vi "Acnetize to ACNET Devices.vi"(8 "error in (no error)":errorcluster, 11 "Acnetize Configuration":string) -> (0 "error out":errorcluster, 3 "ACNET Devices":refnum<class "ACNET Devices.lvclass">)   [LabVIEW 2013]
uses:
  ACNET Monitor/ACNET Devices.lvclass
  ACNET Monitor/ACNET Device.lvclass
  <vilib>/wsapi/NI_WebServices.lvlib
panel:
  out "Array":T1(array[cluster])
  out "subarray":string[](array[string])
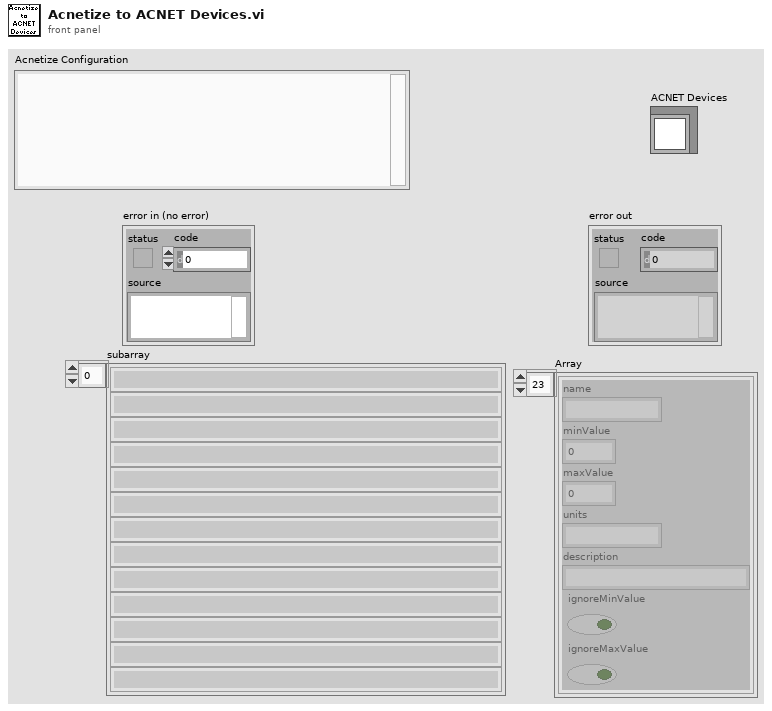
[diagram p1: front panel]
types:
  T1 = cluster{"name":string, "minValue":dbl, "maxValue":dbl, "units":string, "description":string, "ignoreMinValue":bool, "ignoreMaxValue":bool}[]
  T2 = cluster{"name":string, "minValue":dbl, "maxValue":dbl, "units":string, "description":string, "ignoreMinValue":bool, "ignoreMaxValue":bool}
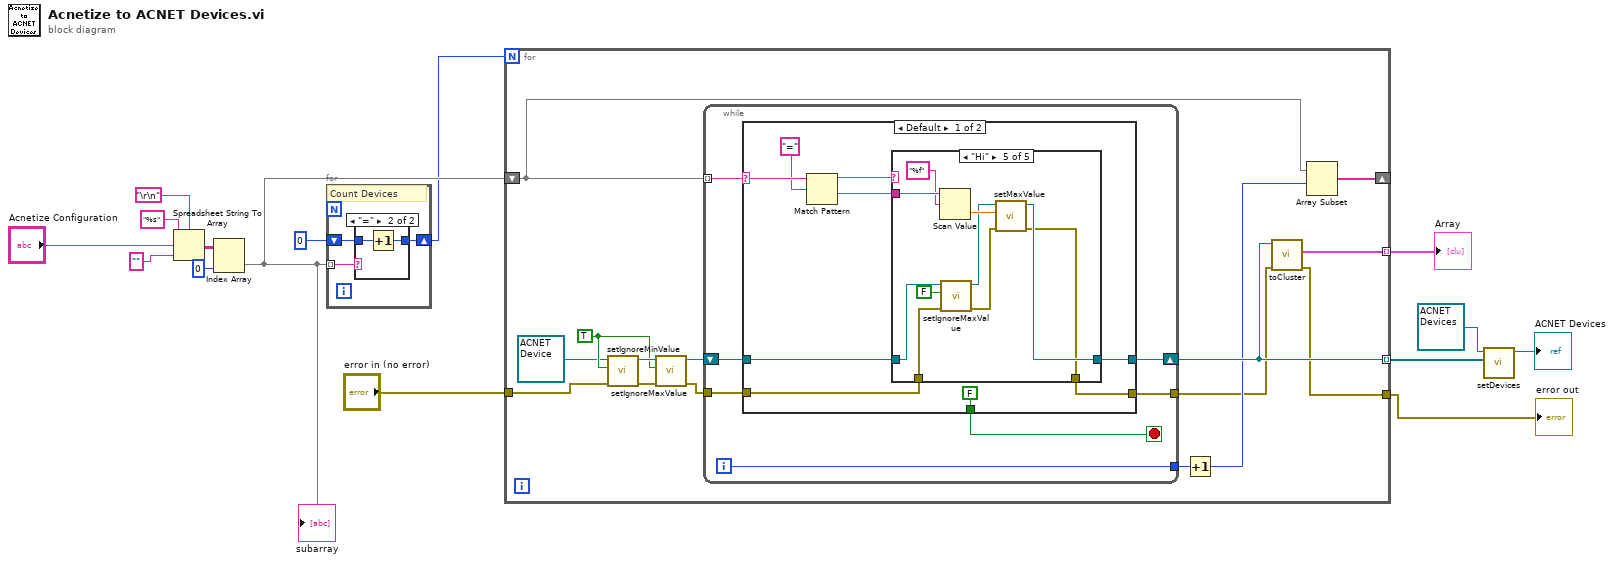
[diagram p0: block diagram]
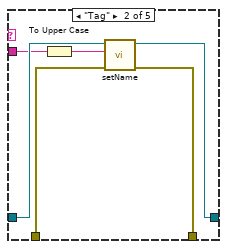
[diagram p3: hidden frame]
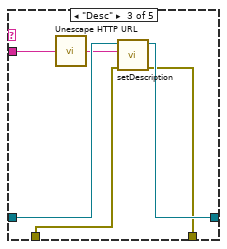
[diagram p4: hidden frame]
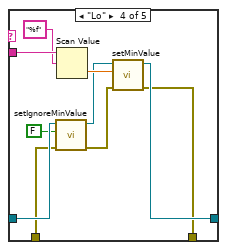
[diagram p5: hidden frame]
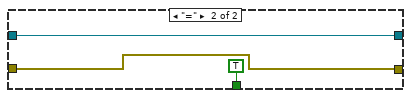
[diagram p6: hidden frame]
diagram:
  n1 = Spreadsheet String To Array(delimiter (Tab)="\r\n", format string="%s", spreadsheet string="Acnetize Configuration", array type (2D Dbl)="") -> (array=w11:string[][])
  n2 = Index Array(array=w11, index (col)=0 ("disabled index (col)")) -> (element=w9:string[])  [unwired: 1 in]
  "subarray" <- w9
  n3 = for {
    tunnel: w9 -> [w18] mode=indexing
    shift-right: [w16] -> w3
    shift-left: 0 -> [w17]
    # "Count Devices"
    n4 = case shown="\"=\"" w18 {
      tunnel: w17 -> [w19 w21]
      tunnel: [w19 w20] -> w16
      frame Default {
      }
      frame "=" {
        n5 = Increment(x=w21) -> (x+1=w20:i32)
      }
    }
  }
  n6 = for {
    N: w3 -> [_]
    tunnel: [w36] -> w7 mode=indexing
    tunnel: [w35] -> w4 mode=indexing
    shift-right: [w31] -> _
    shift-left: w9 -> [w32]
    tunnel: "error in (no error)" -> [w24]
    tunnel: [w29] -> w1
    w26 = TRUE ("ignoreMinValue")
    n7 = call-dynamic "setIgnoreMinValue.vi"("error in (no error)"=w24, "ignoreMinValue"=w26, "ACNET Device in"=refnum<class "ACNET Device.lvclass"> refnum ("ACNET Device.lvclass")) -> ("error out"=w28:errorcluster, "ACNET Device out"=w27:refnum<class "ACNET Device.lvclass">)  [unwired: 7 in]
    n8 = call-dynamic "setIgnoreMaxValue.vi"("error in (no error)"=w28, "ignoreMaxValue"=w26, "ACNET Device in"=w27) -> ("error out"=w23:errorcluster, "ACNET Device out"=w22:refnum<class "ACNET Device.lvclass">)  [unwired: 7 in]
    n9 = while {
      tunnel: w32 -> [w43] mode=indexing
      shift-right: [w41] -> w36
      shift-left: w22 -> [w38]
      tunnel: [w40] -> w34
      tunnel: w23 -> [w37]
      tunnel: [w39] -> w30
      i -> [w40]
      stop <- w42 stop-if-true
      n10 = case shown="Default" w43 {
        selector: w43 -> [w49 _]
        tunnel: [FALSE TRUE] -> w42
        tunnel: w38 -> [w51 w88]
        tunnel: [w50 w88] -> w41
        tunnel: w37 -> [w45 w87]
        tunnel: [w44 w87] -> w39
        frame Default {
          n11 = Match Pattern(string=w49, regular expression="=" ("format string")) -> (before substring=w47:string, after substring=w46:string)  [unwired: 1 in, 2 out]
          n12 = case shown="\"Hi\"" w47 {
            tunnel: w46 -> [_ w56 w64 w75 w85]
            tunnel: w51 -> [w54 w60 w66 w71 w81]
            tunnel: [w54 w59 w65 w76 w86] -> w50
            tunnel: w45 -> [w53 w58 w62 w70 w80]
            tunnel: [w53 w57 w61 w72 w82] -> w44
            frame Default {
            }
            frame "Tag" {
              n13 = To Upper Case(1:w56) -> (0:w55:string)
              n14 = call-dynamic "setName.vi"("error in (no error)"=w58, "name"=w55, "ACNET Device in"=w60) -> ("error out"=w57:errorcluster, "ACNET Device out"=w59:refnum<class "ACNET Device.lvclass">)  [unwired: 7 in]
            }
            frame "Desc" {
              n15 = call <vilib>:"Unescape HTTP URL.vi"("escaped string in"=w64) -> ("unescaped string out"=w63:string)
              n16 = call-dynamic "setDescription.vi"("error in (no error)"=w62, "description"=w63, "ACNET Devices in"=w66) -> ("error out"=w61:errorcluster, "ACNET Devices out"=w65:refnum<class "ACNET Device.lvclass">)  [unwired: 7 in]
            }
            frame "Lo" {
              n17 = call-dynamic "setIgnoreMinValue.vi"("error in (no error)"=w70, "ignoreMinValue"=FALSE, "ACNET Device in"=w71) -> ("error out"=w68:errorcluster, "ACNET Device out"=w69:refnum<class "ACNET Device.lvclass">)  [unwired: 7 in]
              n18 = Scan Value(string=w75, format string="%f") -> (value=w73:dbl)  [unwired: 1 in, 1 out]
              n19 = call-dynamic "setMinValue.vi"("error in (no error)"=w68, "minValue"=w73, "ACNET Devices in"=w69) -> ("error out"=w72:errorcluster, "ACNET Devices out"=w76:refnum<class "ACNET Device.lvclass">)  [unwired: 7 in]
            }
            frame "Hi" {
              n20 = Scan Value(string=w85, format string="%f") -> (value=w83:dbl)  [unwired: 1 in, 1 out]
              n21 = call-dynamic "setIgnoreMaxValue.vi"("error in (no error)"=w80, "ignoreMaxValue"=FALSE, "ACNET Device in"=w81) -> ("error out"=w77:errorcluster, "ACNET Device out"=w78:refnum<class "ACNET Device.lvclass">)  [unwired: 7 in]
              n22 = call-dynamic "setMaxValue.vi"("error in (no error)"=w77, "maxValue"=w83, "ACNET Devices in"=w78) -> ("error out"=w82:errorcluster, "ACNET Devices out"=w86:refnum<class "ACNET Device.lvclass">)  [unwired: 7 in]
            }
          }
        }
        frame "=" {
        }
      }
    }
    n23 = Increment(x=w34) -> (x+1=w33:i32)
    n24 = call-dynamic "toCluster.vi"("error in (no error)"=w30, "ACNET Device in"=w36) -> ("error out"=w29:errorcluster, "ACNET Device Cluster"=w35:T2)  [unwired: 7 in, 1 out]
    n25 = Array Subset(array=w32, index=w33) -> (w31:string[])  [unwired: 1 in]
  }
  "Array" <- w4
  "error out" <- w1
  n26 = call-dynamic "setDevices.vi"("Devices"=w7, "ACNET Devices in"=refnum<class "ACNET Devices.lvclass"> refnum ("ACNET Devices.lvclass")) -> ("ACNET Devices out"=→"ACNET Devices":refnum<class "ACNET Devices.lvclass">)  [unwired: 8 in, 1 out]
